vi "Lectura de documento.vi"() -> ()   [LabVIEW 2023]
panel:
  out "Waveform Chart":dbl[][](graph)
  out "error out 2":errorcluster
  out "error out":errorcluster
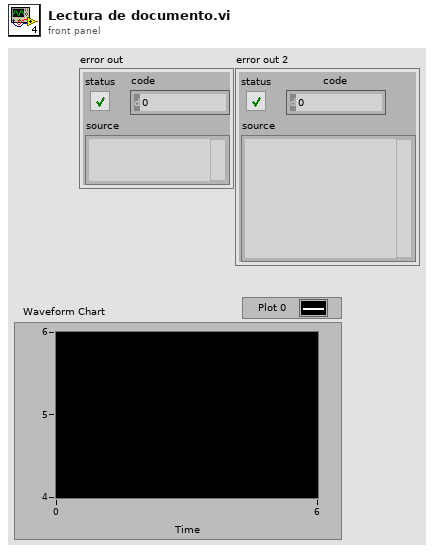
[diagram p1: front panel]
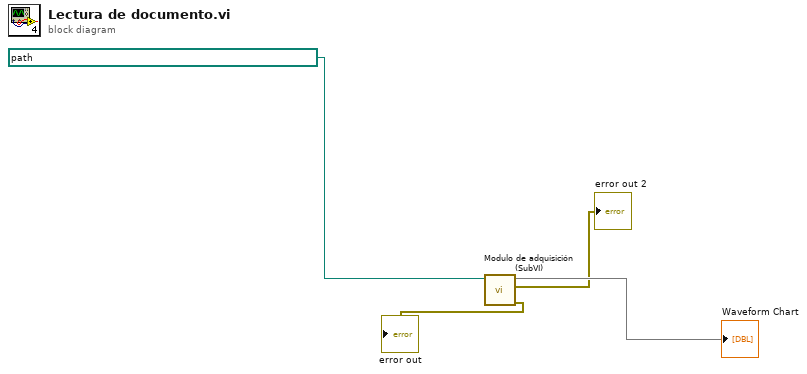
[diagram p0: block diagram]
diagram:
  n1 = call "Modulo de adquisición (SubVI).vi"("file path (use dialog)"=path "C:/Users/chris/Downloads/señal cuadrada.txt") -> ("error out"=→"error out":errorcluster, "error out 2"=→"error out 2":errorcluster, 3:→"Waveform Chart")  [unwired: 8 in]
